vi "BotSpeak_Tiny.vi"(1 "URAPI":string) -> (2 "URAPI  2":string, 3 "SubsString":string, 4 "Tiny Lines":string[](array[string]))   [LabVIEW 2014]
panel:
  in  "Numeric":u8
  # "1st byte - length\n2nd byte - command\n3rd - nth byte values\n\nvalues are 2 bytes each\n\nNumber - is u16 ( hi byte first)\nOtherwise 8 bit source and 8 bit value\nIf MSB = 1, then it is an array\n\nsources:\n\n200 (C8) - TMR[#]\n201 (C9) - AI[#]\n202 (CA) - DIO[#]\n203 (CB) - PWM[#]\n204 (CC) - SERVO[#]\n\n220 (DC) - TMR[var]\n221 (DD) - AI[var]\n222 (DE) - DIO[var]\n223 (DF) - PWM[var]\n224 (E0) - SERVO[var]\n\n252 (FC) - \n253 (FD) - var[var]\n254 (FE) - \n255 (FF) - var#"
  # "a.. abort\nd.. dump\n+ (x2B).. add\n-*/\n\ng (x67)..get\nG (x47)..goto\nI.. (x49) if\n   < x3C\ni.. not if\nP..ping\nr (x72)..run\nd..debug\nR..run and wait\ns (x73)..script\nE (x45).. end script\ne ... go to ScriptSize\n= (x3D)..set\nW (x57)..wait (ms)\nw (x77)..wait (µs)"
  # "DIO 1,1 - raises port 1 high\nDIO 1 - retrieves the status of DIO 1\nSERVO 1,1.5 - sets servo 1 to 1.5 msec (-1 turns off)\nABORT - stops\nDUMP - gives state of all DIO lines in 2 numbers\nAI 0 - replies with value of channel 0\nAO 0,2.5 - sets PWM out to 50%\nSET test,1.2 - sets variable test to 1.2\nGET test - gets value of variable test\nPING - returns version number\nTIMER 1,"
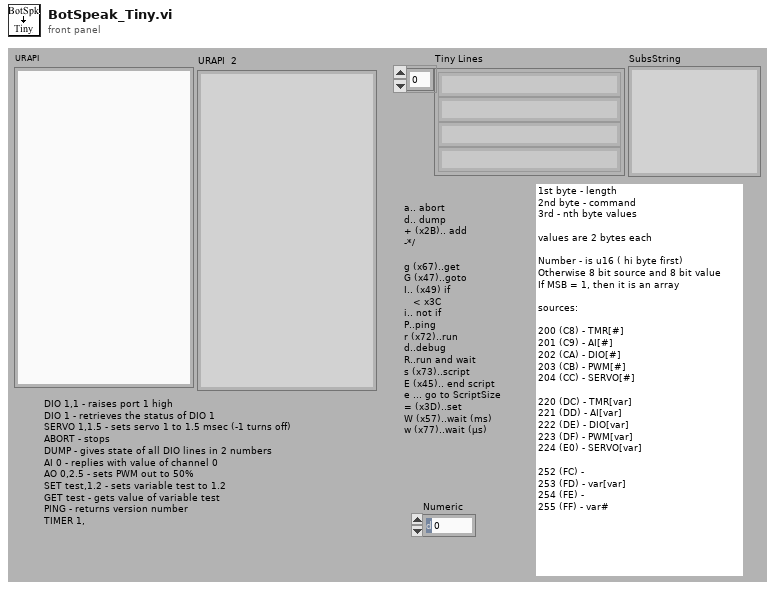
[diagram p1: front panel]
types:
  T1 = cluster{"upper limit":dbl, "lower limit":dbl, "scale":dbl}[]
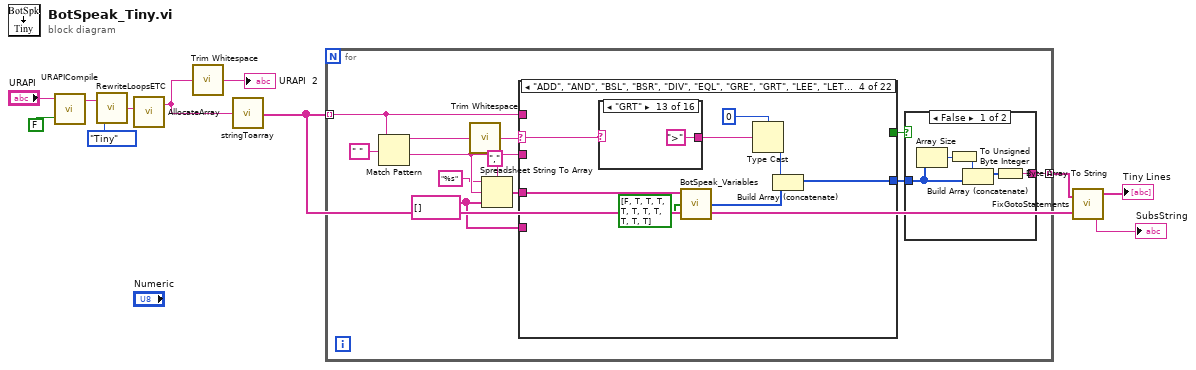
[diagram p0: block diagram]
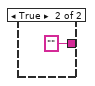
[diagram p2: hidden frame]
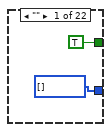
[diagram p3: hidden frame]
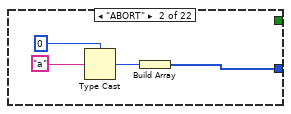
[diagram p4: hidden frame]
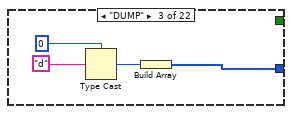
[diagram p5: hidden frame]
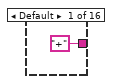
[diagram p6: hidden frame]
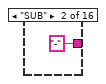
[diagram p7: hidden frame]
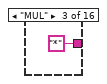
[diagram p8: hidden frame]
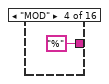
[diagram p9: hidden frame]
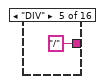
[diagram p10: hidden frame]
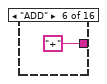
[diagram p11: hidden frame]
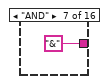
[diagram p12: hidden frame]
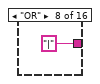
[diagram p13: hidden frame]
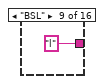
[diagram p14: hidden frame]
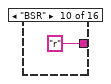
[diagram p15: hidden frame]
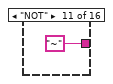
[diagram p16: hidden frame]
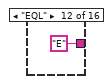
[diagram p17: hidden frame]
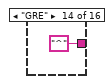
[diagram p18: hidden frame]
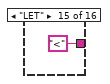
[diagram p19: hidden frame]
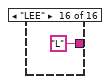
[diagram p20: hidden frame]
diagram:
  n1 = call <userlib>:"URAPICompile.vi"("Comments?"=FALSE, "Script"="URAPI") -> ("trimmed script"=w10:string)
  n2 = call <userlib>:"RewriteLoopsETC.vi"("Type"=enum16{"Tiny", "BotSpeak"}."Tiny", "URAPI in"=w10) -> ("URAPI out"=w6:string)
  n3 = call <userlib>:"AllocateArray.vi"("URAPI in"=w6) -> ("URAPI out"=w5:string)  [unwired: 2 in]
  n4 = call <vilib>:"Trim Whitespace.vi"("string"=w5) -> ("trimmed string"=→"URAPI  2":string)  [unwired: 1 in]
  n5 = call <userlib>:"stringToarray.vi"("String"=w5) -> ("Array"=w4:string[])
  n6 = for {
    tunnel: [w16] -> w8 mode=indexing
    tunnel: w4 -> [w12] mode=indexing
    w14 = string[] []
    n7 = Match Pattern(string=w12, regular expression=" ") -> (before substring=w22:string, after substring=w20:string)  [unwired: 1 in, 2 out]
    n8 = call <vilib>:"Trim Whitespace.vi"("string"=w22) -> ("trimmed string"=w21:string)  [unwired: 1 in]
    n9 = Spreadsheet String To Array(delimiter (Tab)=",", format string="%s", spreadsheet string=w20, array type (2D Dbl)=w14) -> (array=w18:string[])
    n10 = case shown="\"ADD\", \"AND\", \"BSL\", \"BSR\", \"DIV\", \"EQL\", \"GRE\", \"GRT\", \"LEE\", \"LET\", \"MOD\", \"MUL\", \"NOT\", \"OR\", \"SUB\"" w21 {
      selector: w21 -> [_ _ _ w41 _ _ _ _ _ _ _ _ _ _ _ _ _ _ _ _ _ _]
      tunnel: w12 -> [_ _ _ _ _ _ _ _ _ _ _ _ _ _ _ _ _ _ _ _ _ w222]
      tunnel: w20 -> [_ _ _ _ _ _ _ w103 _ _ _ w140 _ _ _ _ _ _ _ _ _ _]
      tunnel: w18 -> [_ _ _ w43 w65 w71 w77 _ _ w119 w125 w134 _ _ w155 w164 w180 w186 w193 w215 w221 _]
      tunnel: [u8[] [] ("unsigned byte array") w32 w36 w45 w66 w72 w78 w104 w115 w120 w126 w141 w145 w149 w156 w168 w181 w188 w198 w217 w220 w223] -> w17
      tunnel: [TRUE _ _ _ _ _ _ _ _ _ _ _ _ _ _ _ _ _ _ _ _ _] -> w15
      tunnel: w14 -> [_ _ _ _ _ _ _ _ _ _ _ _ _ _ _ _ _ _ _ _ _ _]
      frame "" {
      }
      frame "ABORT" {
        n11 = Type Cast(type=u8 0, x="a" ("delimiter (Tab)")) -> (*(type *) &x=w33:u8)
        n12 = Build Array(w33) -> (w32:u8[])
      }
      frame "DUMP" {
        n13 = Type Cast(type=u8 0, x="d" ("delimiter (Tab)")) -> (*(type *) &x=w37:u8)
        n14 = Build Array(w37) -> (w36:u8[])
      }
      frame "ADD", "AND", "BSL", "BSR", "DIV", "EQL", "GRE", "GRT", "LEE", "LET", "MOD", "MUL", "NOT", "OR", "SUB" {
        n15 = case shown="\"GRT\"" w41 {
          tunnel: ["+" ("delimiter (Tab)") "-" ("delimiter (Tab)") "*" ("delimiter (Tab)") "%" ("delimiter (Tab)") "/" ("delimiter (Tab)") "+" ("delimiter (Tab)") "&" ("delimiter (Tab)") "|" ("delimiter (Tab)") "l" ("delimiter (Tab)") "r" ("delimiter (Tab)") "~" ("delimiter (Tab)") "E" ("delimiter (Tab)") ">" ("delimiter (Tab)") "^" ("delimiter (Tab)") "<" ("delimiter (Tab)") "L" ("delimiter (Tab)")] -> w40
          frame Default {
          }
          frame "SUB" {
          }
          frame "MUL" {
          }
          frame "MOD" {
          }
          frame "DIV" {
          }
          frame "ADD" {
          }
          frame "AND" {
          }
          frame "OR" {
          }
          frame "BSL" {
          }
          frame "BSR" {
          }
          frame "NOT" {
          }
          frame "EQL" {
          }
          frame "GRT" {
          }
          frame "GRE" {
          }
          frame "LET" {
          }
          frame "LEE" {
          }
        }
        n16 = call <userlib>:"BotSpeak_Variables.vi"("Var #?"=bool[] [FALSE, TRUE, TRUE, TRUE, TRUE, TRUE, TRUE, TRUE, TRUE, TRUE, TRUE] ("Value of?"), "Variables"=w43) -> ("Binary out"=w46:u8[])  [unwired: 1 in]
        n17 = Type Cast(type=u8 0, x=w40) -> (*(type *) &x=w44:u8)
        n18 = Build Array (concatenate)(w44, w46) -> (w45:u8[])
      }
      frame "GOTO", "goto" {
        n19 = call <userlib>:"BotSpeak_Variables.vi"("Variables"=w65) -> ("Binary out"=w64:u8[])  [unwired: 2 in]
        n20 = Type Cast(type=u8 0, x="G" ("delimiter (Tab)")) -> (*(type *) &x=w67:u8)
        n21 = Build Array (concatenate)(w67, w64) -> (w66:u8[])
      }
      frame "DEBUG" {
        n22 = call <userlib>:"BotSpeak_Variables.vi"("Variables"=w71) -> ("Binary out"=w70:u8[])  [unwired: 2 in]
        n23 = Type Cast(type=u8 0, x="d" ("delimiter (Tab)")) -> (*(type *) &x=w73:u8)
        n24 = Build Array (concatenate)(w73, w70) -> (w72:u8[])
      }
      frame "GOSUB" {
        n25 = call <userlib>:"BotSpeak_Variables.vi"("Variables"=w77) -> ("Binary out"=w76:u8[])  [unwired: 2 in]
        n26 = Type Cast(type=u8 0, x="S" ("delimiter (Tab)")) -> (*(type *) &x=w79:u8)
        n27 = Build Array (concatenate)(w79, w76) -> (w78:u8[])
      }
      frame "IF" {
        w100 = " " ("regular expression")
        w95 = u8 0
        # "will be replaced"
        n28 = Search/Split String(string=w103, search string/char (-)="(" ("regular expression")) -> (substring before match=w90:string, match + rest of string=w85:string)  [unwired: 1 in, 1 out]
        n29 = Search/Split String(string=w85, offset (0)=1) -> (match + rest of string=w83:string)  [unwired: 1 in, 2 out]
        n30 = call <vilib>:"Trim Whitespace.vi"("string"=w90) -> ("trimmed string"=w89:string)  [unwired: 1 in]
        n31 = Match Pattern(string=w83, regular expression=w100) -> (before substring=w96:string, after substring=w101:string)  [unwired: 1 in, 2 out]
        n32 = Match Pattern(string=w101, regular expression=w100) -> (before substring=w94:string, after substring=w99:string)  [unwired: 1 in, 2 out]
        n33 = call <vilib>:"Trim Whitespace.vi"("string"=w94) -> ("trimmed string"=w93:string)  [unwired: 1 in]
        n34 = case shown="\"~\"" w89 {
          tunnel: ["I" ("delimiter (Tab)") "i" ("delimiter (Tab)")] -> w88
          frame Default {
          }
          frame "~" {
          }
        }
        n35 = case shown="\"=\"" w93 {
          tunnel: ["<" ("delimiter (Tab)") "<" ("delimiter (Tab)") ">" ("delimiter (Tab)") "!" ("delimiter (Tab)") "=" ("delimiter (Tab)") "G" ("delimiter (Tab)") "L" ("delimiter (Tab)")] -> w92
          frame Default {
          }
          frame "<" {
          }
          frame ">" {
          }
          frame "!=", "<>" {
          }
          frame "=" {
          }
          frame ">=" {
          }
          frame "<=" {
          }
        }
        n36 = Match Pattern(string=w99, regular expression=")") -> (before substring=w97:string)  [unwired: 1 in, 3 out]
        n37 = Build Array(w96, w97, "0" ("regular expression")) -> (w87:string[])
        n38 = Type Cast(type=w95, x=w92) -> (*(type *) &x=w91:u8)
        n39 = Type Cast(type=w95, x=w88) -> (*(type *) &x=w105:u8)
        n40 = call <userlib>:"BotSpeak_Variables.vi"("Variables"=w87) -> ("Binary out"=w86:u8[])  [unwired: 2 in]
        n41 = Build Array (concatenate)(w105, w91, w86) -> (w104:u8[])
      }
      frame "PING" {
        n42 = Type Cast(type=u8 0, x="P" ("delimiter (Tab)")) -> (*(type *) &x=w116:u8)
        n43 = Build Array(w116) -> (w115:u8[])
      }
      frame "RUN" {
        n44 = call <userlib>:"BotSpeak_Variables.vi"("Variables"=w119) -> ("Binary out"=w121:u8[])  [unwired: 2 in]
        n45 = Type Cast(type=u8 0, x="r" ("delimiter (Tab)")) -> (*(type *) &x=w122:u8)
        n46 = Build Array (concatenate)(w122, w121) -> (w120:u8[])
      }
      frame "RUN&WAIT" {
        n47 = call <userlib>:"BotSpeak_Variables.vi"("Variables"=w125) -> ("Binary out"=w127:u8[])  [unwired: 2 in]
        n48 = Type Cast(type=u8 0, x="R" ("delimiter (Tab)")) -> (*(type *) &x=w128:u8)
        n49 = Build Array (concatenate)(w128, w127) -> (w126:u8[])
      }
      frame "SCRIPT" {
        n50 = Match Pattern(string=w140, regular expression="," ("delimiter (Tab)")) -> (after substring=w136:string)  [unwired: 1 in, 3 out]
        n51 = Match Pattern(string=w136, regular expression="," ("delimiter (Tab)")) -> (after substring=w135:string)  [unwired: 1 in, 3 out]
        n52 = Array Subset(array=w134, length=2) -> (w132:string[])  [unwired: 1 in]
        n53 = call <userlib>:"BotSpeak_Variables.vi"("Variables"=w132) -> ("Binary out"=w131:u8[])  [unwired: 2 in]
        n54 = String To Byte Array(string=w135) -> (unsigned byte array=w138:u8[])
        n55 = Type Cast(type=u8 0, x="s" ("delimiter (Tab)")) -> (*(type *) &x=w142:u8)
        n56 = Build Array (concatenate)(w142, w131, w138) -> (w141:u8[])
      }
      frame "ENDSCRIPT" {
        n57 = Type Cast(type=u8 0, x="E" ("delimiter (Tab)")) -> (*(type *) &x=w146:u8)
        n58 = Build Array(w146) -> (w145:u8[])
      }
      frame "END", "end" {
        n59 = Type Cast(type=u8 0, x="e" ("delimiter (Tab)")) -> (*(type *) &x=w150:u8)
        n60 = Build Array(w150) -> (w149:u8[])
      }
      frame "SERVO" {
        n61 = Type Cast(type=u8 0, x="S" ("delimiter (Tab)")) -> (*(type *) &x=w157:u8)
        n62 = call <userlib>:"BotSpeak_Variables.vi"("Scaling"=T1 [{"upper limit"=0.0, "lower limit"=0.0, "scale"=0.0}, {"upper limit"=3.0, "lower limit"=0.0, "scale"=180.0}], "Variables"=w155) -> ("Binary out"=w153:u8[])  [unwired: 1 in]
        n63 = Build Array (concatenate)(w157, w153) -> (w156:u8[])
      }
      frame "SET" {
        n64 = Index Array(array=w164) -> (element=w163:string)  [unwired: 1 in]
        n65 = Match Pattern(string=w163, regular expression="\\[") -> (before substring=w161:string)  [unwired: 1 in, 3 out]
        n66 = case shown="Default" w161 {
          tunnel: [T1 [{"upper limit"=0.0, "lower limit"=0.0, "scale"=1.0}, {"upper limit"=0.0, "lower limit"=0.0, "scale"=1.0}, {"upper limit"=0.0, "lower limit"=0.0, "scale"=1.0}, {"upper limit"=0.0, "lower limit"=0.0, "scale"=1.0}, {"upper limit"=0.0, "lower limit"=0.0, "scale"=1.0}, {"upper limit"=0.0, "lower limit"=0.0, "scale"=1.0}, {"upper limit"=0.0, "lower limit"=0.0, "scale"=1.0}, {"upper limit"=0.0, "lower limit"=0.0, "scale"=1.0}, {"upper limit"=0.0, "lower limit"=0.0, "scale"=1.0}, {"upper limit"=0.0, "lower limit"=0.0, "scale"=1.0}, {"upper limit"=0.0, "lower limit"=0.0, "scale"=1.0}] ("Scaling") T1 [{"upper limit"=1.0, "lower limit"=0.0, "scale"=1.0}, {"upper limit"=100.0, "lower limit"=0.0, "scale"=100.0}, {"upper limit"=1.0, "lower limit"=0.0, "scale"=1.0}, {"upper limit"=0.0, "lower limit"=0.0, "scale"=1.0}, {"upper limit"=0.0, "lower limit"=0.0, "scale"=1.0}, {"upper limit"=0.0, "lower limit"=0.0, "scale"=1.0}, {"upper limit"=0.0, "lower limit"=0.0, "scale"=1.0}, {"upper limit"=0.0, "lower limit"=0.0, "scale"=1.0}, {"upper limit"=0.0, "lower limit"=0.0, "scale"=1.0}, {"upper limit"=0.0, "lower limit"=0.0, "scale"=1.0}, {"upper limit"=0.0, "lower limit"=0.0, "scale"=1.0}] ("Scaling") T1 [{"upper limit"=1.0, "lower limit"=0.0, "scale"=1.0}, {"upper limit"=2.0, "lower limit"=1.0, "scale"=100.0}, {"upper limit"=0.0, "lower limit"=0.0, "scale"=1.0}, {"upper limit"=0.0, "lower limit"=0.0, "scale"=1.0}, {"upper limit"=0.0, "lower limit"=0.0, "scale"=1.0}, {"upper limit"=0.0, "lower limit"=0.0, "scale"=1.0}, {"upper limit"=0.0, "lower limit"=0.0, "scale"=1.0}, {"upper limit"=0.0, "lower limit"=0.0, "scale"=1.0}, {"upper limit"=0.0, "lower limit"=0.0, "scale"=1.0}, {"upper limit"=0.0, "lower limit"=0.0, "scale"=1.0}, {"upper limit"=0.0, "lower limit"=0.0, "scale"=1.0}] ("Scaling") T1 [{"upper limit"=0.0, "lower limit"=0.0, "scale"=1.0}, {"upper limit"=1.0, "lower limit"=0.0, "scale"=1.0}, {"upper limit"=0.0, "lower limit"=0.0, "scale"=1.0}, {"upper limit"=0.0, "lower limit"=0.0, "scale"=1.0}, {"upper limit"=0.0, "lower limit"=0.0, "scale"=1.0}, {"upper limit"=0.0, "lower limit"=0.0, "scale"=1.0}, {"upper limit"=0.0, "lower limit"=0.0, "scale"=1.0}, {"upper limit"=0.0, "lower limit"=0.0, "scale"=1.0}, {"upper limit"=0.0, "lower limit"=0.0, "scale"=1.0}, {"upper limit"=0.0, "lower limit"=0.0, "scale"=1.0}, {"upper limit"=0.0, "lower limit"=0.0, "scale"=1.0}] ("Scaling")] -> w160
          frame Default {
          }
          frame "PWM" {
          }
          frame "SERVO" {
          }
          frame "DIO" {
          }
        }
        n67 = Type Cast(type=u8 0, x="=" ("delimiter (Tab)")) -> (*(type *) &x=w167:u8)
        n68 = call <userlib>:"BotSpeak_Variables.vi"("Scaling"=w160, "Var #?"=bool[] [TRUE, TRUE, TRUE, TRUE, TRUE, TRUE, TRUE, TRUE, TRUE, TRUE, TRUE] ("Value of?"), "Variables"=w164) -> ("Binary out"=w165:u8[])
        n69 = Build Array (concatenate)(w167, w165) -> (w168:u8[])
      }
      frame "SYSTEM" {
        n70 = call <userlib>:"BotSpeak_Variables.vi"("Var #?"=bool[] [TRUE, TRUE, TRUE, TRUE, TRUE, TRUE, TRUE, TRUE, TRUE, TRUE, TRUE] ("Value of?"), "Variables"=w180) -> ("Binary out"=w177:u8[])  [unwired: 1 in]
        n71 = Array Size(array=w177) -> (size(s)=w176:i32)
        n72 = Type Cast(type=u8 0, x="!" ("delimiter (Tab)")) -> (*(type *) &x=w178:u8)
        n73 = To Unsigned Byte Integer(number=w176) -> (unsigned 8bit integer=w175:u8)
        n74 = Build Array (concatenate)(w178, w175, w177) -> (w181:u8[])
      }
      frame "GET" {
        n75 = Type Cast(type=u8 0, x="g" ("delimiter (Tab)")) -> (*(type *) &x=w187:u8)
        n76 = call <userlib>:"BotSpeak_Variables.vi"("Var #?"=bool[] [TRUE, TRUE, TRUE, TRUE, TRUE, TRUE, TRUE, TRUE, TRUE, TRUE, TRUE] ("Value of?"), "Variables"=w186) -> ("Binary out"=w184:u8[])  [unwired: 1 in]
        n77 = Build Array (concatenate)(w187, w184) -> (w188:u8[])
      }
      frame "WAIT" {
        n78 = Index Array(array=w193) -> (element=w196:string)  [unwired: 1 in]
        n79 = Scan From String(input string=w196) -> (error out=w195:errorcluster, output 1=w194:dbl)  [unwired: 4 in, 2 out]
        n80 = case shown="No Error" w195 {
          tunnel: [w202 "W" ("delimiter (Tab)")] -> w197
          tunnel: w194 -> [w206 _]
          tunnel: w193 -> [_ _]
          tunnel: [w201 T1 [{"upper limit"=0.0, "lower limit"=0.0, "scale"=1.0}] ("Scaling")] -> w191
          frame No Error {
            n81 = Absolute Value(x=w206) -> (abs(x)=w205:dbl)
            n82 = Less?(x=w205, y=0.01) -> (x < y?=w203:bool)
            n83 = case shown="True" w203 {
              tunnel: ["w" ("delimiter (Tab)") "W" ("delimiter (Tab)")] -> w202
              tunnel: [T1 [{"upper limit"=0.0, "lower limit"=0.0, "scale"=1000000.0}] ("Scaling") T1 [{"upper limit"=0.0, "lower limit"=0.0, "scale"=1000.0}] ("Scaling")] -> w201
              frame True {
              }
              frame False {
              }
            }
          }
          frame Error {
            # "variable for wait time\n(in msec)"
          }
        }
        n84 = Type Cast(type=u8 0, x=w197) -> (*(type *) &x=w199:u8)
        n85 = call <userlib>:"BotSpeak_Variables.vi"("Scaling"=w191, "Variables"=w193) -> ("Binary out"=w192:u8[])  [unwired: 1 in]
        n86 = Build Array (concatenate)(w199, w192) -> (w198:u8[])
      }
      frame "WAITµs" {
        n87 = call <userlib>:"BotSpeak_Variables.vi"("Scaling"=T1 [{"upper limit"=0.0, "lower limit"=0.0, "scale"=1.0}], "Variables"=w215) -> ("Binary out"=w213:u8[])  [unwired: 1 in]
        n88 = Type Cast(type=u8 0, x="w" ("delimiter (Tab)")) -> (*(type *) &x=w218:u8)
        n89 = Build Array (concatenate)(w218, w213) -> (w217:u8[])
      }
      frame "convert" {
        n90 = call <userlib>:"BotSpeak_Variables.vi"("Variables"=w221) -> ("Binary out"=w220:u8[])  [unwired: 2 in]
      }
      frame Default {
        n91 = String To Byte Array(string=w222) -> (unsigned byte array=w223:u8[])
      }
    }
    n92 = case shown="False" w15 {
      tunnel: w17 -> [w26 _]
      tunnel: [w28 "" ("string")] -> w16
      frame False {
        n93 = Array Size(array=w26) -> (size(s)=w27:i32)
        n94 = To Unsigned Byte Integer(number=w27) -> (unsigned 8bit integer=w24:u8)
        n95 = Build Array (concatenate)(w24, w26) -> (w25:u8[])
        n96 = Byte Array To String(unsigned byte array=w25) -> (string=w28:string)
      }
      frame True {
      }
    }
  }
  n97 = call <userlib>:"FixGotoStatements.vi"("URAPI LInes"=w4, "Tiny Lines"=w8) -> ("SubsString"=→"SubsString":string, "Tiny Fixed"=→"Tiny Lines":string[])  [unwired: 1 out]
